vi "DAQmx Write (Digital Bool 1Line 1Point).vi"(8 "error in":errorcluster, 11 "task in":refnum<class "Session Factory.lvclass">) -> (0 "error out":errorcluster, 3 "task out":refnum<class "Session Factory.lvclass">)   [LabVIEW 2021, in "Session Management niDAQmx.lvlib" / "Session Factory.lvclass"]
uses:
  Session Factory.lvclass
  Session Factory.lvclass/Session Factory.ctl
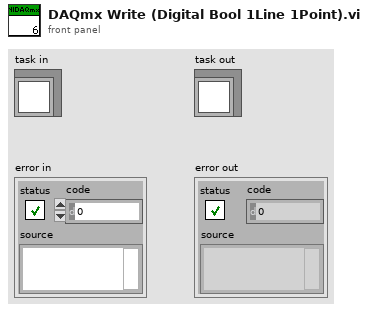
[diagram p1: front panel]
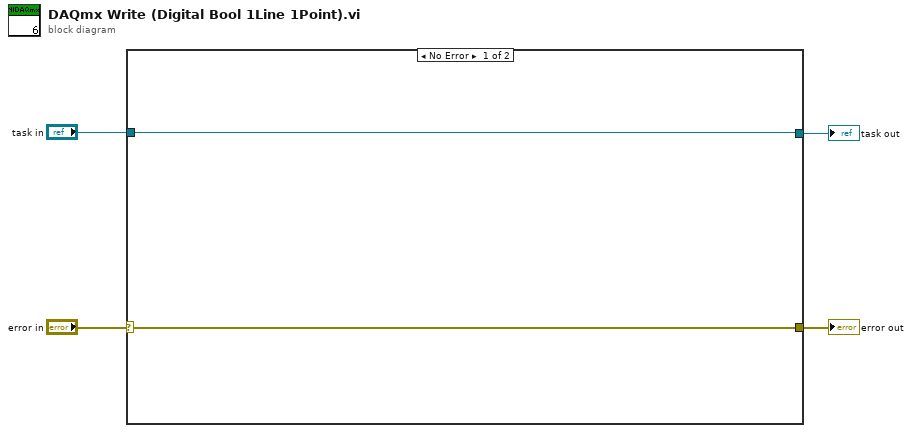
[diagram p0: block diagram]
diagram:
  n1 = case shown="No Error" "error in" {
    selector: "error in" -> [w6 w8]
    tunnel: [w6 w8] -> w3
    tunnel: "task in" -> [w5 w7]
    tunnel: [w5 w7] -> w1
    frame No Error {
    }
    frame Error {
    }
  }
  "error out" <- w3
  "task out" <- w1
